vi "dual gate sts.vi"() -> ()   [LabVIEW 2021]
panel:
  in  "Tabs":enum32{"Main", "Attributes"}(tab)
  in  "Safety Limit 2 (V)":dbl
  in  "Basename":string
  in  "Start Gate 2 (V)":dbl
  in  "End Gate 2 (V)":dbl
  in  "Increment Gate 2 (V)":dbl
  in  "Stop":bool
  out "Current Gate Voltage 2 (V)":dbl
  in  "Attributes":string[][](array[string])
  # "Dual Gate STS"
  # "Gate 2 Parameters"
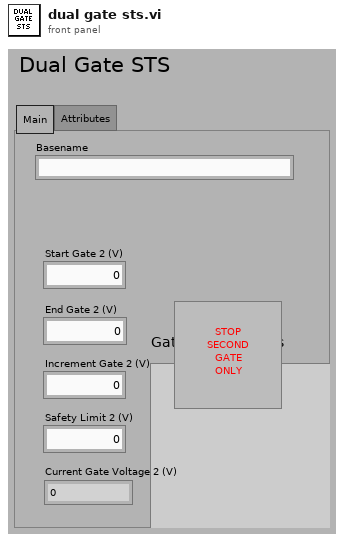
[diagram p1: front panel]
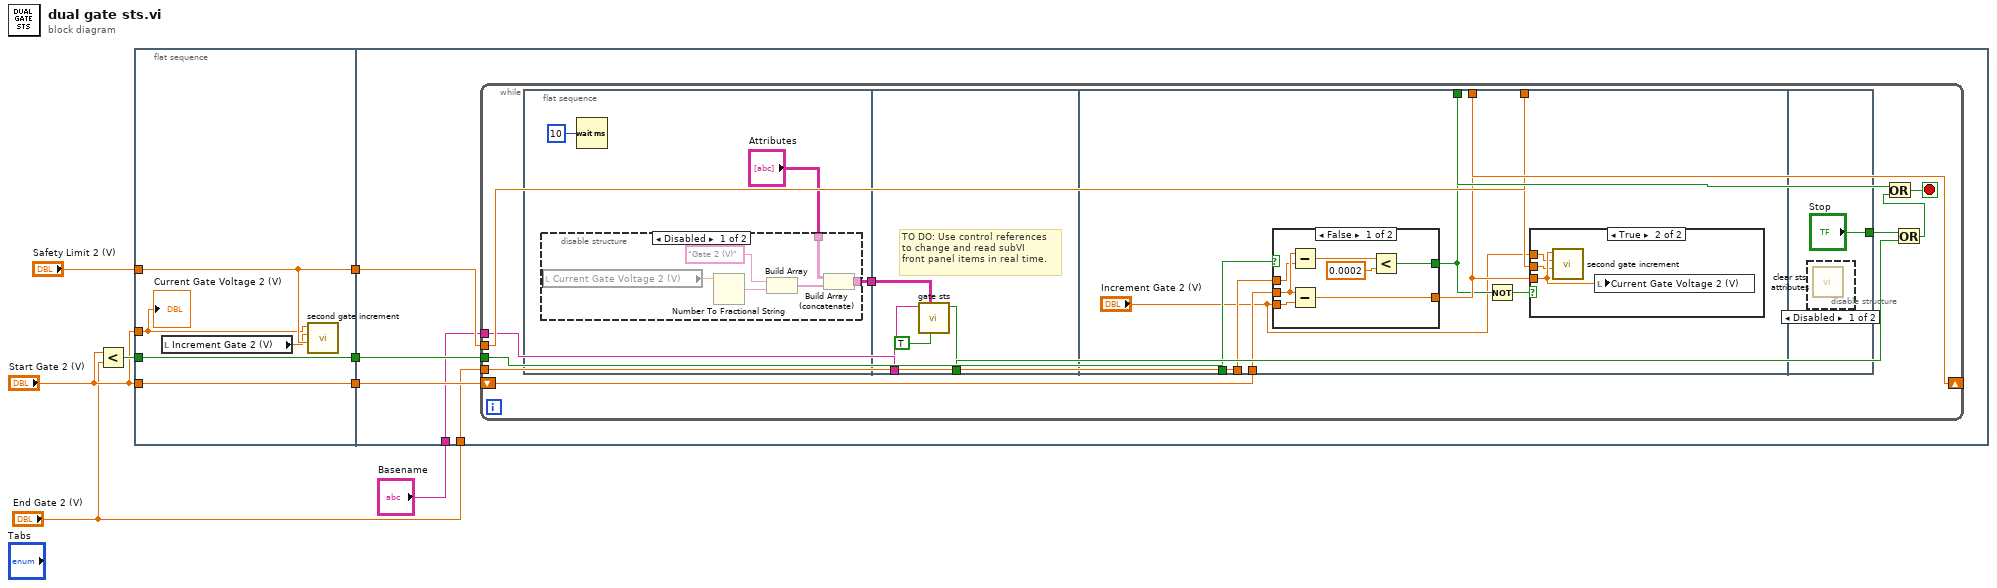
[diagram p0: block diagram]
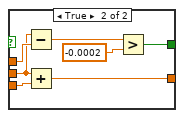
[diagram p3: hidden frame]
diagram:
  n1 = Less?(x="Start Gate 2 (V)", y="End Gate 2 (V)") -> (x < y?=w8:bool)
  n2 = flat-sequence {
    tunnel: [w13] -> w4
    tunnel: [w12] -> w3
    tunnel: [w11] -> w2
    tunnel: "Safety Limit 2 (V)" -> [w11]
    tunnel: "Start Gate 2 (V)" -> [w10]
    tunnel: "Start Gate 2 (V)" -> [w12]
    tunnel: w8 -> [w13]
    tunnel: w4 -> [w18]
    tunnel: w3 -> [w17]
    tunnel: "End Gate 2 (V)" -> [w16]
    tunnel: w2 -> [w15]
    tunnel: "Basename" -> [w14]
    frame #0 {
      n3 = local read "Increment Gate 2 (V)"() -> (w9:dbl)
      n4 = call "second gate increment.vi"("Voltage Safety Limit"=w11, "Increment"=w9, "Gate Voltage"=w10) -> ()  [unwired: 9 in]
      "Current Gate Voltage 2 (V)" <- w10
    }
    frame #1 {
      n5 = while {
        tunnel: w18 -> [w25]
        shift-right: [w29] -> _
        shift-left: w17 -> [w27]
        tunnel: w16 -> [w26]
        tunnel: w15 -> [w24]
        tunnel: w14 -> [w23]
        stop <- w30 stop-if-true
        n6 = flat-sequence {
          tunnel: [w31] -> w22
          tunnel: w23 -> [w43]
          tunnel: w22 -> [w44]
          tunnel: [w42] -> w21
          tunnel: [w52] -> w29
          tunnel: [w51] -> w28
          tunnel: w27 -> [w50]
          tunnel: w26 -> [w49]
          tunnel: w25 -> [w48]
          tunnel: w24 -> [w46]
          tunnel: ["Stop"] -> w19
          frame #0 {
            n7 = disable-structure shown="Disabled" {
              disable-tunnel: "Attributes" -> [w37 w40]
              disable-tunnel: [w34 w40] -> w31
              frame Disabled {
                n8 = local read "Current Gate Voltage 2 (V)"() -> (w38:dbl)
                n9 = Number To Fractional String(number=w38) -> (F-format string=w39:string)  [unwired: 3 in]
                n10 = Build Array("Gate 2 (V)" ("element"), w39) -> (w36:string[])
                n11 = Build Array (concatenate)(w37, w36) -> (w34:string[][])
              }
              frame Enabled {
              }
            }
            n12 = Wait (ms)(milliseconds to wait=u32 10) -> ()  [unwired: 1 out]
          }
          frame #1 {
            # "TO DO: Use control references\nto change and read subVI\nfront panel items in real time."
            n13 = call "gate sts.vi"("Store\nSecond Gate?"=TRUE ("Store\nSecond Gate?"), "Attributes"=w44, "Basename"=w43) -> ("Stop Loop"=w42:bool)  [unwired: 7 in]
          }
          frame #2 {
            n14 = case shown="False" w48 {
              tunnel: w50 -> [w57 w63]
              tunnel: "Increment Gate 2 (V)" -> [w58 w66]
              tunnel: [w59 w65] -> w52
              tunnel: w49 -> [w56 w64]
              tunnel: [w54 w62] -> w51
              frame False {
                n15 = Subtract(x=w57, y=w56) -> (x-y=w55:dbl)
                n16 = Subtract(x=w57, y=w58) -> (x-y=w59:dbl)
                n17 = Less?(x=w55, y=0.0002) -> (x < y?=w54:bool)
              }
              frame True {
                n18 = Subtract(x=w63, y=w64) -> (x-y=w61:dbl)
                n19 = Add(x=w63, y=w66) -> (x+y=w65:dbl)
                n20 = Greater?(x=w61, y=-0.0002) -> (0:w62:bool)
              }
            }
            n21 = Not(x=w51) -> (.not. x?=w47:bool)
            n22 = case shown="True" w47 {
              tunnel: w52 -> [_ w69]
              tunnel: w46 -> [_ w68]
              tunnel: "Increment Gate 2 (V)" -> [_ w67]
              frame False {
              }
              frame True {
                n23 = call "second gate increment.vi"("Voltage Safety Limit"=w68, "Increment"=w67, "Gate Voltage"=w69) -> ()  [unwired: 9 in]
                n24 = local write "Current Gate Voltage 2 (V)"(w69) -> ()
              }
            }
          }
          frame #3 {
            n25 = disable-structure shown="Disabled" {
              frame Disabled {
                n26 = call "clear sts attributes.vi"() -> ()  [unwired: 12 in]
              }
              frame Enabled {
              }
            }
          }
        }
        n27 = Or(x=w19, y=w21) -> (x .or. y?=w20:bool)
        n28 = Or(x=w28, y=w20) -> (x .or. y?=w30:bool)
      }
    }
  }
